vi "Initialize Error Log.vi"(8 "error in (no error)":errorcluster, 11 "Error Handler In":refnum<class "Error Handler.lvclass">) -> (0 "error out":errorcluster, 3 "Error Handler Out":refnum<class "Error Handler.lvclass">)   [LabVIEW 2020, in "Error Handler.lvclass"]
uses:
  Error Handler.lvclass
  C:/Users/anton/Documents/GitHub/LUnit/source/Application Framework/Process Classes/Process/Process.lvclass
  Process/Process.lvclass/Process.ctl
  Error Handler.lvclass/Error Handler.ctl
  Support/Error Log Classes/Text Log/Text Log.lvclass
  C:/Users/anton/Documents/GitHub/LUnit/source/Application Framework/Support/Error Log Classes/Error Log/Error Log.lvclass
  C:/Users/anton/Documents/GitHub/LUnit/source/Application Framework/Support/Error Log Classes/Text Log/Text Log.lvclass
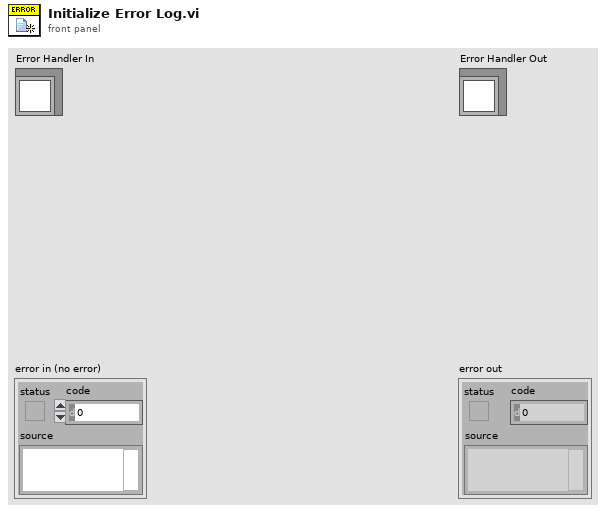
[diagram p1: front panel]
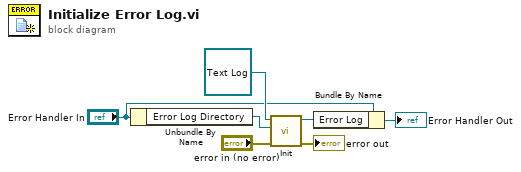
[diagram p0: block diagram]
diagram:
  n1 = Unbundle By Name("Error Handler In") -> ("Error Log Directory"=w4:path)
  n2 = call-dynamic "Init.vi"("error in (no error)"="error in (no error)", "Error Log Path"=w4, "Text Log in"=refnum<class "Text Log.lvclass"> refnum ("Error Log Classes.lvlib:Text Log.lvclass")) -> ("error out"=→"error out":errorcluster, "Text Log out"=w6:refnum<class "Text Log.lvclass">)  [unwired: 7 in]
  n3 = Bundle By Name(cluster="Error Handler In", "Error Log"=w6) -> (→"Error Handler Out":refnum<class "Error Handler.lvclass">)
